vi "countphotons.vi"(0 "Gating Counter":tag="Dev1/ctr2" caption="Counter(s)", 6 "error in":errorcluster, 8 "Initial delay (ms)":dbl format="%.2f", 9 "Count time (ms)":dbl=1.0 caption="High Time (seconds)" format="%0.2f", 10 "Input Counter 2":tag="Dev1/ctr1" caption="Counter(s)", 11 "Input Counter 1":tag="Dev1/ctr0" caption="Counter(s)") -> (2 "Pulses Counted 2":u32 caption="Data", 3 "Pulses Counted":u32 caption="Data", 4 "error out":errorcluster)   [LabVIEW 2013]
doc: "I. Description:\nThis example demonstrates how to count digital events on a Counter Input Channel. The Initial Count, Count Direction, and Edge are all configurable. \n\nEdges are counted on the counter's default input terminal (refer to section IV, I/O Connections Overview, below for more information), but could easily be modified to count edges on a PFI or RTSI line.\n\nII. Instructions for Running:\n1. Select the Physical Channel which corresponds to the counter you want to count edges on the DAQ device.\n2. Enter the Initial Count, Count Direction, and measurement Edge to specify how you want the counter to count. Additionally, you can change the input terminal where events are counted using the channel property node.\nNote: Use the Gen Dig Pulse Train-Continuous example to verify that you are counting correctly on the DAQ device.\n\nIII. Block Diagram Steps:\n1. Create a Counter Input channel to Count Events. The Edge parameter is used to determine if the counter will increment on rising or falling edges.\n2. Call the Start VI to arm the counter and begin counting. The counter will be preloaded with the Initial Count.\n3. The counter will be continually polled until the Stop button is pressed on the front panel.\n4. Call the Clear Task VI to clear the Task.\n5. Use the popup dialog box to display an error if any.\n\nIV. I/O Connections Overview:\nThe counter will count edges on the input terminal of the counter specified in the Physical Channel I/O control.\n\nIn this example the counter will count edges on the default input terminal on ctr0.\n\nFor more information on the default counter input and output terminals for your device, open the NI-DAQmx Help, and refer to Counter Signal Connections found under the Device Considerations book in the table of contents."
uses:
  <vilib>/Utility/error.llb/DialogType.ctl
  <vilib>/DAQmx/read.llb/DAQmx Read (Counter U32 1Chan 1Samp).vi
  <vilib>/DAQmx/create/channels.llb/DAQmx Create Channel (CI-Count Edges).vi
  <vilib>/DAQmx/create/channels.llb/DAQmx Create Channel (CO-Pulse Generation-Time).vi
  <vilib>/DAQmx/configure/events/hardwareSignals.llb/DAQmx Export Signal (Most Signals).vi
  <vilib>/DAQmx/miscellaneous.llb/DAQmx Fill In Error Info.vi
  <resource>/objmgr/daqmx.rc
panel:
  # "INPUTS"
  # "OUTPUT"
  # "Specify two counters on the DAQ\ncard to count pulses."
  # "Specify a different counter on the DAQ card which will be used internally to set the length of the counting time. (This counter is only used for timing and doesn't actually count anything, so it can be any counter which isn't being used as Input Counter 1 or 2.)"
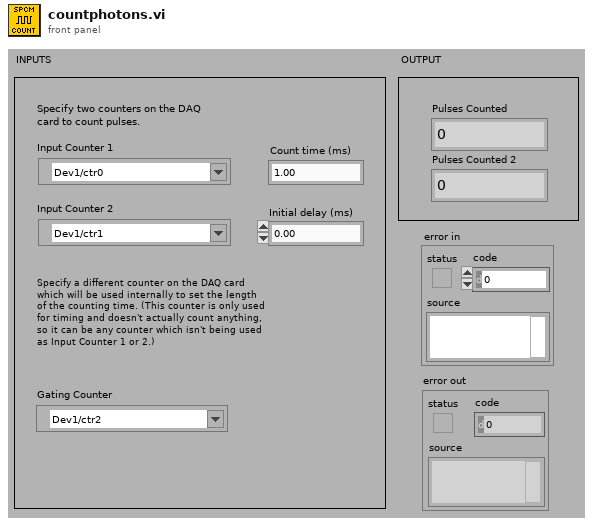
[diagram p1: front panel]
types:
  T1 = typedef "DialogType.ctl" = u16
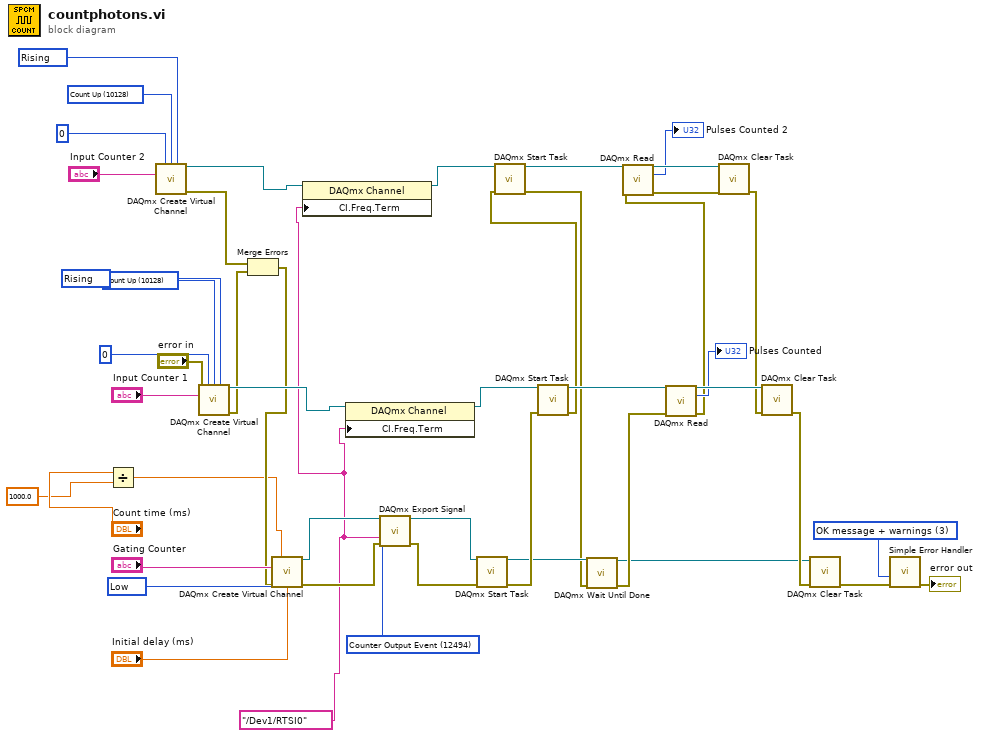
[diagram p0: block diagram]
diagram:
  w20 = 10128 items=["Count Up"=10128, "Count Down"=10124, "Externally Controlled"=10326] ("Count Direction")
  w21 = 10280 items=["Rising"=10280, "Falling"=10171] ("Edge")
  w36 = 10214 items=["High"=10192, "Low"=10214] ("Idle State")
  w40 = 10128 items=["Count Up"=10128, "Count Down"=10124, "Externally Controlled"=10326] ("Count Direction")
  w41 = 10280 items=["Rising"=10280, "Falling"=10171] ("Edge")
  w26 = 12494 items=["AI Convert Clock"=12484, "10MHz Reference Clock"=12536, "20MHz Timebase Clock"=12486, "Sample Clock"=12487, "Advance Trigger"=12488, "Reference Trigger"=12490, "Start Trigger"=12491, "Advance Complete Event"=12492, "AI Hold Complete Event"=12493, "Counter Output Event"=12494, "Change Detection Event"=12511, "Watchdog Timer Expired Event"=12512] ("signal")
  w14 = tag "/Dev1/RTSI0" ("output terminal")
  w34 = T1 3 items=["no dialog", "OK message", "continue or stop message", "OK message + warnings", "continue/stop + warnings"] ("type of dialog (OK msg:1)")
  n1 = Divide(x="Count time (ms)", y=1000.0) -> (x/y=w5:dbl)
  n2 = call-poly <vilib>:"DAQmx Create Virtual Channel.vi"("initial count"=u32 0 ("Initial Count"), "count direction"=w20, "edge"=w21, "counter"="Input Counter 2") -> ("task out"=w15:refnum<k21>, "error out"=w8:errorcluster)  [unwired: 10 in]
  n3 = call-poly <vilib>:"DAQmx Create Virtual Channel.vi"("initial count"=u32 0 ("Initial Count"), "count direction"=w40, "edge"=w41, "counter"="Input Counter 1", "error in"="error in") -> ("task out"=w24:refnum<k21>, "error out"=w7:errorcluster)  [unwired: 9 in]
  n4 = Merge Errors(w8, w7) -> (w6:errorcluster)
  n5 = call-poly <vilib>:"DAQmx Create Virtual Channel.vi"("high time"=w5, "counter"="Gating Counter", "error in"=w6, "idle state"=w36, "initial delay"="Initial delay (ms)") -> ("task out"=w30:refnum<k21>, "error out"=w29:errorcluster)  [unwired: 9 in]
  n6 = property class="DAQmx Channel"(reference=w15, "CI.Freq.Term"=w14) -> (reference out=w16:refnum<k21>)  [unwired: 1 in, 1 out]
  n7 = property class="DAQmx Channel"(reference=w24, "CI.Freq.Term"=w14) -> (reference out=w25:refnum<k21>)  [unwired: 1 in, 1 out]
  n8 = call-poly <vilib>:"DAQmx Export Signal.vi"("task/channels in"=w30, "signal"=w26, "output terminal"=w14, "error in"=w29) -> ("task out"=w27:refnum<k21>, "error out"=w28:errorcluster)  [unwired: 10 in]
  n9 = call <vilib>:"DAQmx Start Task.vi"("task/channels in"=w27, "error in"=w28) -> ("task out"=w32:refnum<k21>, "error out"=w44:errorcluster)  [unwired: 12 in]
  n10 = call <vilib>:"DAQmx Start Task.vi"("task/channels in"=w25, "error in"=w44) -> ("task out"=w33:refnum<k21>, "error out"=w13:errorcluster)  [unwired: 12 in]
  n11 = call <vilib>:"DAQmx Start Task.vi"("task/channels in"=w16, "error in"=w13) -> ("task out"=w17:refnum<k21>, "error out"=w12:errorcluster)  [unwired: 12 in]
  n12 = call <vilib>:"DAQmx Wait Until Done.vi"("task/channels in"=w32, "error in"=w12) -> ("task out"=w31:refnum<k21>, "error out"=w38:errorcluster)  [unwired: 12 in]
  n13 = call-poly <vilib>:"DAQmx Read.vi"("task/channels in"=w33, "error in"=w38) -> ("task out"=w47:refnum<k21>, "data"=→"Pulses Counted":u32, "error out"=w11:errorcluster)  [unwired: 11 in]
  n14 = call-poly <vilib>:"DAQmx Read.vi"("task/channels in"=w17, "error in"=w11) -> ("task out"=w23:refnum<k21>, "data"=→"Pulses Counted 2":u32, "error out"=w10:errorcluster)  [unwired: 11 in]
  n15 = call <vilib>:"DAQmx Clear Task.vi"("task in"=w23, "error in"=w10) -> ("error out"=w9:errorcluster)  [unwired: 13 in]
  n16 = call <vilib>:"DAQmx Clear Task.vi"("task in"=w47, "error in"=w9) -> ("error out"=w43:errorcluster)  [unwired: 13 in]
  n17 = call <vilib>:"DAQmx Clear Task.vi"("task in"=w31, "error in"=w43) -> ("error out"=w42:errorcluster)  [unwired: 13 in]
  n18 = call <vilib>:"Simple Error Handler.vi"("type of dialog (OK msg:1)"=w34, "error in (no error)"=w42) -> ("error out"=→"error out":errorcluster)  [unwired: 3 in, 4 out]
